vi "Templates get www-templates Folder.vi"(3 "Relative Path (\"\")":string) -> (1 "WWW-templates Folder":path)   [LabVIEW 2011]
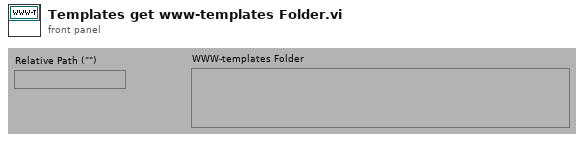
[diagram p1: front panel]
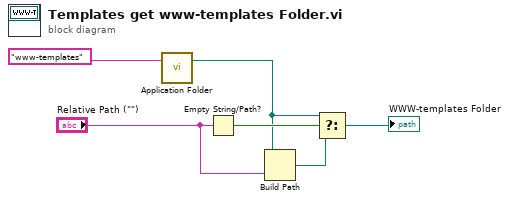
[diagram p0: block diagram]
diagram:
  n1 = call "Application Folder.vi"("Relative Path (\"\" - Folder)"="www-templates" ("name or relative path")) -> ("Application Folder"=w2:path)  [unwired: 2 in]
  n2 = Empty String/Path?(string/path="Relative Path (\"\")") -> (empty?=w5:bool)
  n3 = Build Path(base path=w2, name or relative path="Relative Path (\"\")") -> (appended path=w3:path)
  n4 = Select(t=w2, s=w5, f=w3) -> (s? t:f=→"WWW-templates Folder":path)
